vi "runViComplexNode.vi"(8 "error in (no error)":errorcluster) -> (0 "error out":errorcluster, 3 "variantOut":variant)   [LabVIEW 2018]
doc: "Run the vi wil the complex inputs and outputs by the node."
uses:
  src/VariantTool/getValFromVariant_double.vi
panel:
  out "data":dbl
  in  "imag":dbl
  in  "real":dbl
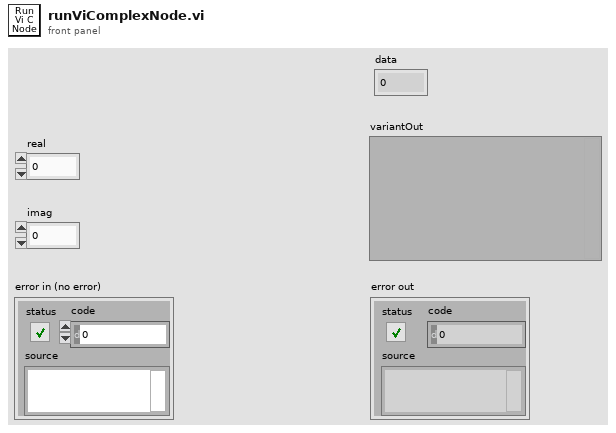
[diagram p1: front panel]
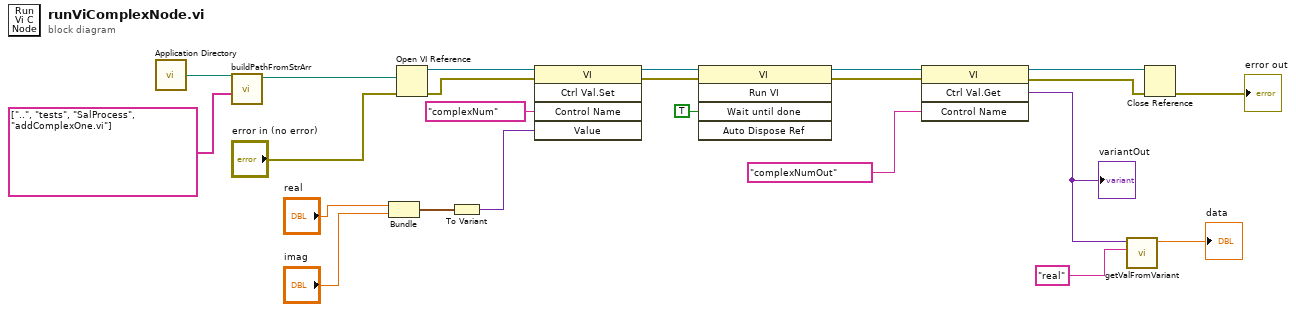
[diagram p0: block diagram]
diagram:
  n1 = call <vilib>:"Application Directory.vi"() -> ("Application Directory"=w23:path)
  n2 = call "buildPathFromStrArr.vi"("String Array"=string[] ["..", "tests", "SalProcess", "addComplexOne.vi"], "Root Path"=w23) -> ("Absolute Path"=w21:path)  [unwired: 9 in]
  n3 = Bundle("real"="real", "imag"="imag") -> (w5:cluster{"real":dbl, "imag":dbl})  [unwired: 1 in]
  n4 = Open VI Reference(vi path=w21, error in (no error)="error in (no error)") -> (vi reference=w18:refnum<vi>, error out=w17:errorcluster)  [unwired: 4 in]
  n5 = To Variant(anything=w5) -> (Variant=w4:variant)
  n6 = invoke class="VI" method="Ctrl Val.Set"(reference=w18, error in=w17, "Control Name"="complexNum", "Value"=w4) -> (reference out=w16:refnum<vi>, error out=w15:errorcluster)  [unwired: 1 in, 3 out]
  n7 = invoke class="VI" method="Run VI"(reference=w16, error in=w15, "Wait until done"=TRUE ("Wait Until Done")) -> (reference out=w13:refnum<vi>, error out=w12:errorcluster)  [unwired: 2 in, 3 out]
  n8 = invoke class="VI" method="Ctrl Val.Get"(reference=w13, error in=w12, "Control Name"="complexNumOut") -> (reference out=w11:refnum<vi>, error out=w6:errorcluster, "Get Control Value Variant"=w2:variant)  [unwired: 1 in, 1 out]
  "variantOut" <- w2
  n9 = call-poly "getValFromVariant.vi"("name"="real", "variant"=w2) -> ("value"=→"data":dbl)  [unwired: 8 in, 1 out]
  n10 = Close Reference(reference=w11, error in (no error)=w6) -> (error out=→"error out":errorcluster)
